vi "Create Edge Map.vi"(8 "error in (no error)":errorcluster, 10 "Keyed Edge to Detect":refnum<class "1D Array s64.lvclass">, 11 "Is Value Below Treshold?":refnum<class "2D Array binary.lvclass">) -> (0 "error out":errorcluster, 3 "Edge Map":refnum<class "2D Array binary.lvclass">)   [LabVIEW 2020, in "G2CPU Line Profile.lvlib"]
uses:
  G2CPU Line Profile.lvlib
  <vilib>/Natan Biesmans/G2CPU GPU and CPU HPC Toolkit/G2CPU Libraries/Arrays/1DArray/s64/1D Array s64.lvclass
  C:/Program Files/National Instruments/LabVIEW 2025/vi.lib/Natan Biesmans/G2CPU GPU and CPU HPC Toolkit/G2CPU Libraries/Arrays/Array/Array Prototype.lvclass
  <vilib>/Natan Biesmans/G2CPU GPU and CPU HPC Toolkit/G2CPU Libraries/Arrays/2DArray/binary/2D Array binary.lvclass
  <vilib>/Natan Biesmans/G2CPU GPU and CPU HPC Toolkit/G2CPU Libraries/Arrays/Array/Array Prototype.lvclass/Array Prototype.ctl
  e203accf-83b4-452c-bbba-4048955b1189.vi
  7d1bd0df-84a8-41fd-ac1a-d0ac994ef2be.vi
  07d4b031-b753-4afc-ae6c-e53d66100d9e.vi
  82d3cdf1-c825-4bc7-884e-549f3b69fcfa.vi
  f258b7ca-8cdf-4dfa-a800-a64dc1b66162.vi
  5572ab95-9b47-47af-b2fc-01c2c1a17515.vi
  6150ca03-74eb-4a5f-b4db-82e702bfa66c.vi
  <vilib>/Natan Biesmans/G2CPU GPU and CPU HPC Toolkit/G2CPU Libraries/Arrays/Array/G2CPU Get Array Pointer.vi
  e203accf-83b4-452c-bbba-4048955b1189.vi/e7247370-a01f-465a-ac0e-4dfefcb1bb87.vi
  e203accf-83b4-452c-bbba-4048955b1189.vi/345e91f0-9a5e-4de4-af9c-133346717e4a.vi
  7d1bd0df-84a8-41fd-ac1a-d0ac994ef2be.vi/08cb2c43-1c8b-4a3a-83bc-b3e8cdef0e3a.vi
  7d1bd0df-84a8-41fd-ac1a-d0ac994ef2be.vi/f755307d-5806-43cd-9fa2-5ac75ab59def.vi
  7d1bd0df-84a8-41fd-ac1a-d0ac994ef2be.vi/37397dd5-2c89-4701-b050-64d2f1e61e81.vi
  07d4b031-b753-4afc-ae6c-e53d66100d9e.vi/cfed8f62-9c64-4dab-912e-5e7c21cb720b.vi
  82d3cdf1-c825-4bc7-884e-549f3b69fcfa.vi/e9bebd79-1c27-4fc1-b91f-30516104c7f0.vi
  f258b7ca-8cdf-4dfa-a800-a64dc1b66162.vi/5793b77b-c002-4ebf-9075-685617c95341.vi
  f258b7ca-8cdf-4dfa-a800-a64dc1b66162.vi/2ed3ef86-c00d-4d71-b84c-20267a6dfcf9.vi
  5572ab95-9b47-47af-b2fc-01c2c1a17515.vi/e9bebd79-1c27-4fc1-b91f-30516104c7f0.vi
  6150ca03-74eb-4a5f-b4db-82e702bfa66c.vi/e2b7cdad-9748-47a9-8803-19dad6ab3e2b.vi
  6150ca03-74eb-4a5f-b4db-82e702bfa66c.vi/edeb7e37-ba5b-4522-b7cc-59d3333e22dd.vi
  07d4b031-b753-4afc-ae6c-e53d66100d9e.vi/cfed8f62-9c64-4dab-912e-5e7c21cb720b.vi/77c7badc-ed81-4514-99c1-20d37f4e5ecc.vi
  07d4b031-b753-4afc-ae6c-e53d66100d9e.vi/cfed8f62-9c64-4dab-912e-5e7c21cb720b.vi/eb76fa01-6782-47b4-b34f-9eb474c9cc78.vi
  <vilib>/Natan Biesmans/G2CPU GPU and CPU HPC Toolkit/ArrayFire Driver/VIs/Run as Multi Device.vi
  f258b7ca-8cdf-4dfa-a800-a64dc1b66162.vi/5793b77b-c002-4ebf-9075-685617c95341.vi/3e802c67-fb96-46a3-ae13-4994a8508b4f.vi
  f258b7ca-8cdf-4dfa-a800-a64dc1b66162.vi/5793b77b-c002-4ebf-9075-685617c95341.vi/5a50fc67-79e7-4972-80c2-92243cd53dd4.vi
  f258b7ca-8cdf-4dfa-a800-a64dc1b66162.vi/2ed3ef86-c00d-4d71-b84c-20267a6dfcf9.vi/730f6c57-5c0b-4ee9-b61e-75067b25222b.vi
  f258b7ca-8cdf-4dfa-a800-a64dc1b66162.vi/2ed3ef86-c00d-4d71-b84c-20267a6dfcf9.vi/096b8799-7810-404e-baca-ba9279cec4bd.vi
  f258b7ca-8cdf-4dfa-a800-a64dc1b66162.vi/2ed3ef86-c00d-4d71-b84c-20267a6dfcf9.vi/0f1a5a47-bcc5-4796-ac31-8dfcfbc0d7d1.vi
  f258b7ca-8cdf-4dfa-a800-a64dc1b66162.vi/2ed3ef86-c00d-4d71-b84c-20267a6dfcf9.vi/89f12e17-3330-4b72-ad8f-8dd636660732.vi
  6150ca03-74eb-4a5f-b4db-82e702bfa66c.vi/e2b7cdad-9748-47a9-8803-19dad6ab3e2b.vi/edd31282-7992-4bba-af75-482693dee5e1.vi
  <vilib>/Natan Biesmans/G2CPU GPU and CPU HPC Toolkit/G2CPU Libraries/Arrays/2DArray/s64/2D Array s64.lvclass
  <vilib>/Natan Biesmans/G2CPU GPU and CPU HPC Toolkit/ArrayFire Driver/VIs/cast.vi
  <vilib>/Natan Biesmans/G2CPU GPU and CPU HPC Toolkit/G2CPU Libraries/Arrays/Array/G2CPU Set Array Pointer.vi
  <vilib>/Natan Biesmans/G2CPU GPU and CPU HPC Toolkit/G2CPU Libraries/Arrays/Array/G2CPU Release Array.vi
  <vilib>/Natan Biesmans/G2CPU GPU and CPU HPC Toolkit/ArrayFire Driver/VIs/diff1.vi
  <vilib>/Natan Biesmans/G2CPU GPU and CPU HPC Toolkit/ArrayFire Driver/VIs/iszero.vi
  <vilib>/Natan Biesmans/G2CPU GPU and CPU HPC Toolkit/ArrayFire Driver/VIs/sub.vi
  <vilib>/Natan Biesmans/G2CPU GPU and CPU HPC Toolkit/ArrayFire Driver/VIs/release array.vi
  <vilib>/Natan Biesmans/G2CPU GPU and CPU HPC Toolkit/ArrayFire Driver/subvi/Error Converter (ErrCode or Status).vi
  <vilib>/Natan Biesmans/G2CPU GPU and CPU HPC Toolkit/ArrayFire Driver/VIs/add.vi
  <vilib>/Natan Biesmans/G2CPU GPU and CPU HPC Toolkit/ArrayFire Driver/VIs/transpose.vi
  <vilib>/Natan Biesmans/G2CPU GPU and CPU HPC Toolkit/G2CPU Libraries/Arrays/SubVI/is 2D.vi
  <vilib>/Natan Biesmans/G2CPU GPU and CPU HPC Toolkit/ArrayFire Driver/VIs/eq.vi
  <vilib>/Natan Biesmans/G2CPU GPU and CPU HPC Toolkit/G2CPU Libraries/Arrays/Array/Array Prototype.lvclass
  <vilib>/Natan Biesmans/G2CPU GPU and CPU HPC Toolkit/G2CPU Libraries/Arrays/2DArray/2D Array Prototype.lvclass
  <vilib>/Natan Biesmans/G2CPU GPU and CPU HPC Toolkit/G2CPU Libraries/Arrays/DataTypes/I64/s64.lvclass
  <vilib>/Natan Biesmans/G2CPU GPU and CPU HPC Toolkit/G2CPU Libraries/Arrays/1DArray/1D Array Prototype.lvclass
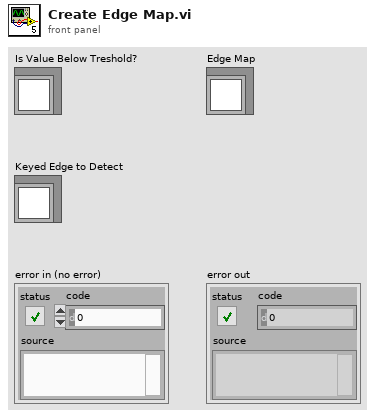
[diagram p1: front panel]
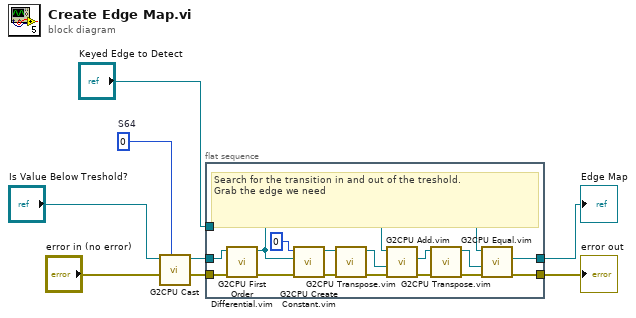
[diagram p0: block diagram]
diagram:
  w1 = i64 0  # S64
  n1 = call "G2CPU Cast"("Datatype Prototype"=w1, "error in (no error)"="error in (no error)", "Array In"="Is Value Below Treshold?") -> ("error out"=w4:errorcluster, "Array Out"=w5:refnum<class "2D Array s64.lvclass">)  [unwired: 7 in]
  n2 = flat-sequence {
    tunnel: [w24] -> w2
    tunnel: [w23] -> w3
    tunnel: "Keyed Edge to Detect" -> [w18]
    tunnel: w4 -> [w22]
    tunnel: w5 -> [w21]
    frame #0 {
      # "Search for the transition in and out of the treshold.\nGrab the edge we need"
      n3 = call "G2CPU First Order Differential.vim"("error in (no error)"=w22, "Array in"=w21) -> ("error out"=w20:errorcluster, "Array Result"=w17:refnum<class "2D Array s64.lvclass">)  [unwired: 8 in]
      n4 = call "G2CPU Create Constant.vim"("error in (no error)"=w20, "Size"=w17, "val"=i64 0) -> ("error out"=w12:errorcluster, "object out"=w16:refnum<class "2D Array s64.lvclass">)  [unwired: 7 in]
      n5 = call "G2CPU Transpose.vim"("error in (no error)"=w12, "Array In"=w16) -> ("error out"=w11:errorcluster, "Array out"=w15:refnum<class "2D Array s64.lvclass">)  [unwired: 8 in]
      n6 = call "G2CPU Add.vim"("error in (no error)"=w11, "Array rhs"=w15, "Array lhs"=w18) -> ("error out"=w10:errorcluster, "Array Result"=w14:refnum<class "2D Array s64.lvclass">)  [unwired: 7 in]
      n7 = call "G2CPU Transpose.vim"("error in (no error)"=w10, "Array In"=w14) -> ("error out"=w9:errorcluster, "Array out"=w13:refnum<class "2D Array s64.lvclass">)  [unwired: 8 in]
      n8 = call "G2CPU Equal.vim"("error in (no error)"=w9, "Array rhs"=w13, "Array lhs"=w17) -> ("error out"=w24:errorcluster, "Array Result"=w23:refnum<class "2D Array binary.lvclass">)  [unwired: 7 in]
    }
  }
  "Edge Map" <- w3
  "error out" <- w2
